vi "TDMS - AeroQuad File Viewer.vi"(4 "error in (no error)":errorcluster, 7 "file path":path) -> (0 "error out":errorcluster, 3 "file path out":path)   [LabVIEW 2010]
doc: "Opens the .tdms file specified in the <B>file path</B> input and presents the file data in the TDMS File Viewer dialog box."
uses:
  <vilib>/Utility/tdmsutil.llb/fileViewerConfigData.ctl
  <vilib>/Utility/error.llb/DialogType.ctl
  <vilib>/Utility/tdmsutil.llb/TDMSFileViewerLocalizedText.vi
  Instance           1 26Saved   TDMS - File Viewer .vi
panel:
  in  "Help":bool
  in  "Status":string
  in  "Quit":bool
  in  "Settings...":bool
  in  "Properties / Values / Graph":T1(tab)
  in  "Properties":i32(listbox)
  in  "Raw data values":i32(listbox)
  out "Waveform Graph":waveform(dbl)[](graph)
  in  "File contents":string(tree)
  # "Displaying values 1..1000"
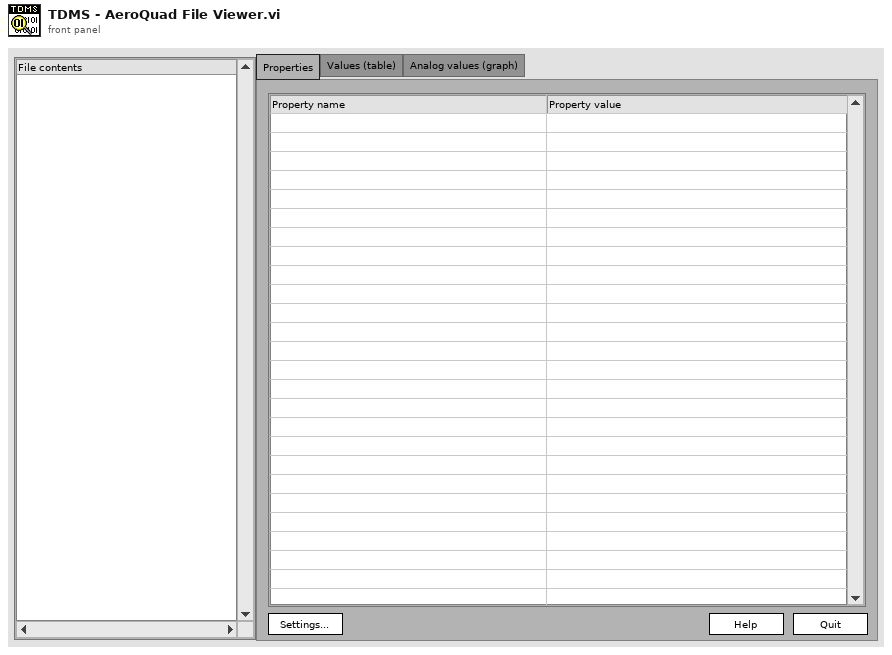
[diagram p1: front panel]
types:
  T1 = enum32{"Properties", "Values (table)", "Analog values (graph)"}
  T2 = enum16{"open", "open or create", "create or replace", "create", "open (read-only)"}
  T3 = typedef "fileViewerConfigData.ctl" = cluster{"Show all (table)":bool, "Show all (graph)":bool, "limit (table)":u64, "limit (graph)":u64, "no show":bool, "start (table)":u64, "start (graph)":u64}
  T4 = cluster{"Tree":refnum<vi>, "Tab Control":refnum<vi>, "property list":refnum<vi>, "raw data list":refnum<vi>, "Waveform Graph":refnum<vi>, "Ok":refnum<vi>, "Ok 2":refnum<vi>, "Ok 3":refnum<vi>, "Ok 4":refnum<vi>}
  T5 = typedef "LVRectTypeDef.ctl" = cluster{"left":i16, "top":i16, "right":i16, "bottom":i16}
  T6 = typedef "DialogType.ctl" = u16
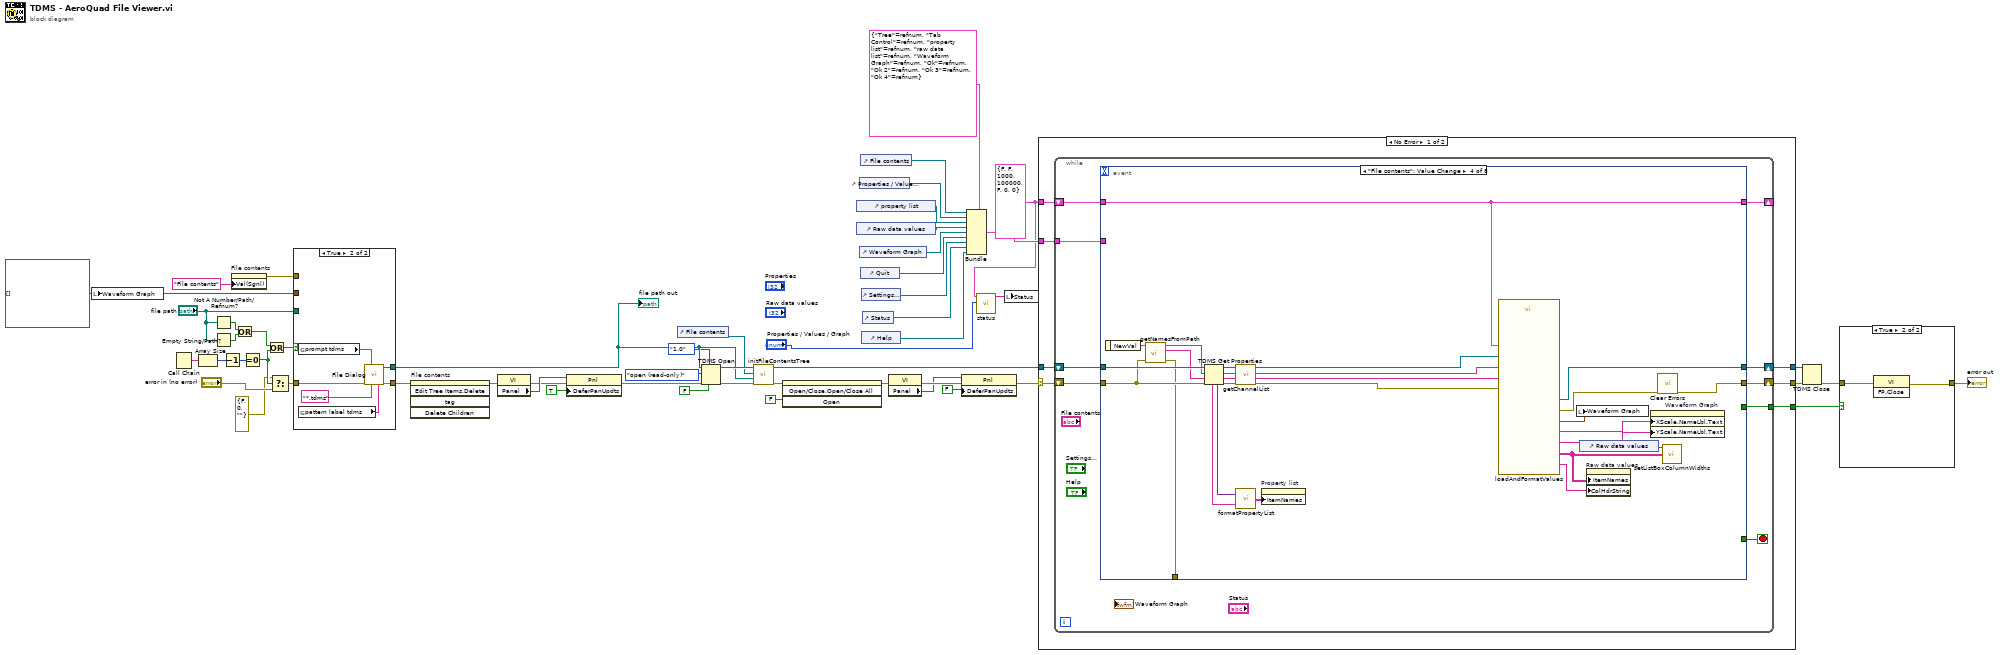
[diagram p0: block diagram]
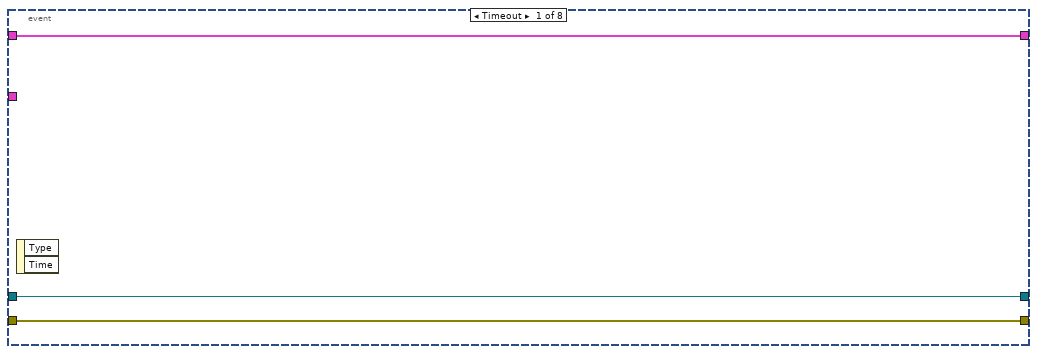
[diagram p3: hidden frame]
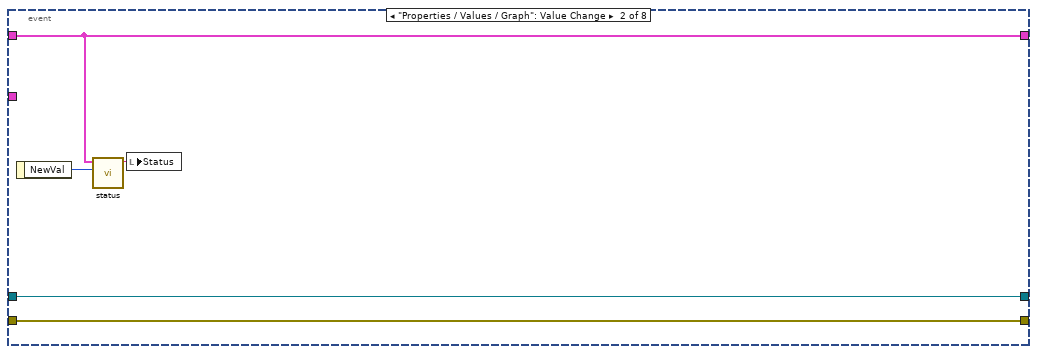
[diagram p4: hidden frame]
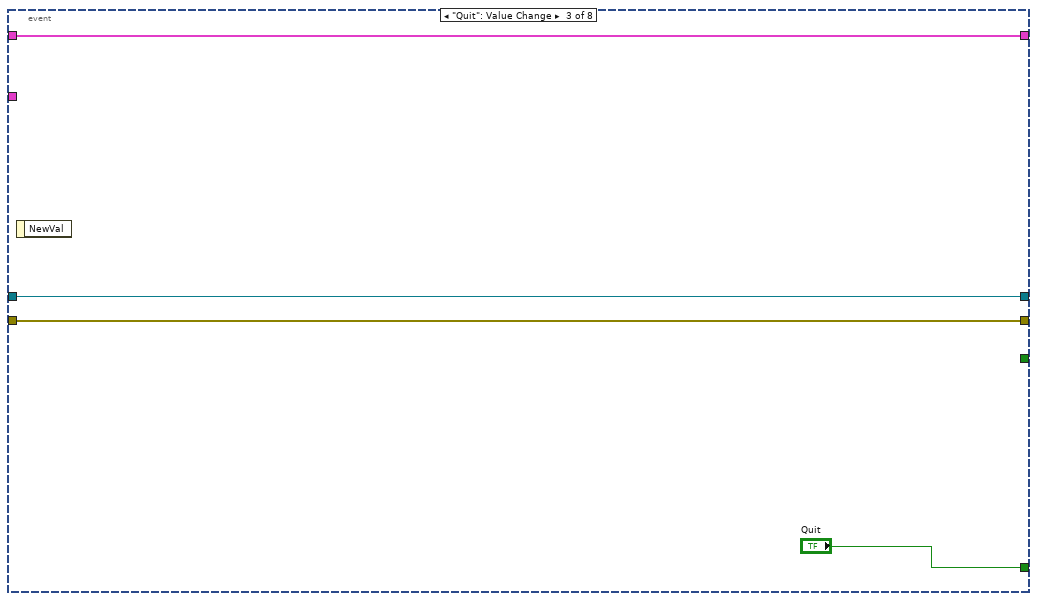
[diagram p5: hidden frame]
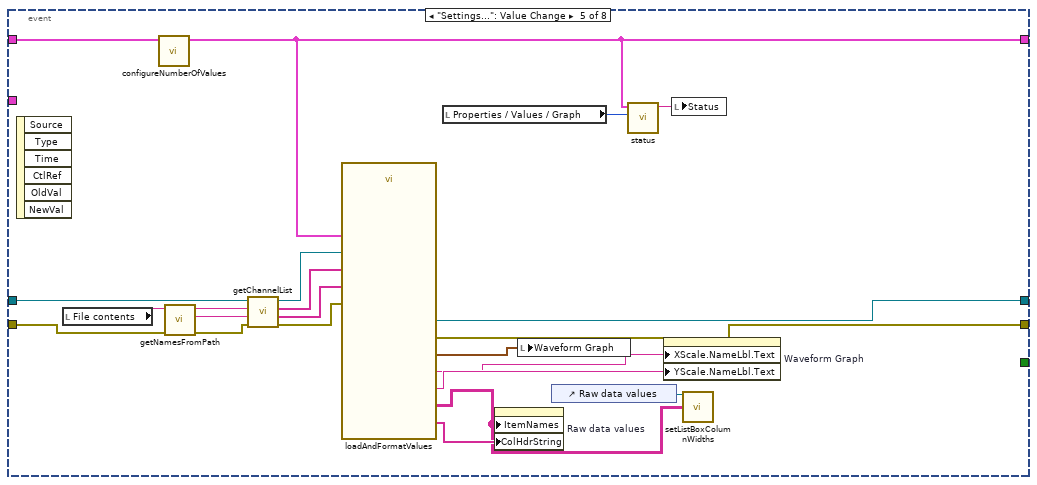
[diagram p6: hidden frame]
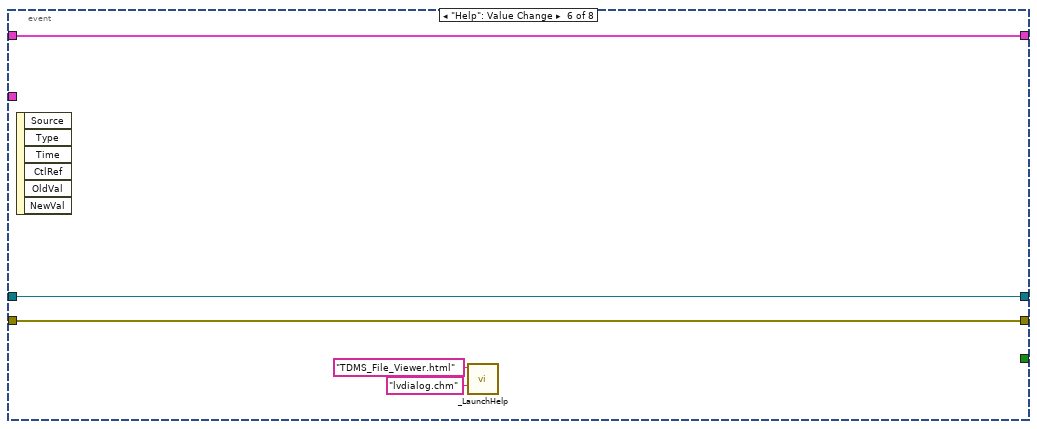
[diagram p7: hidden frame]
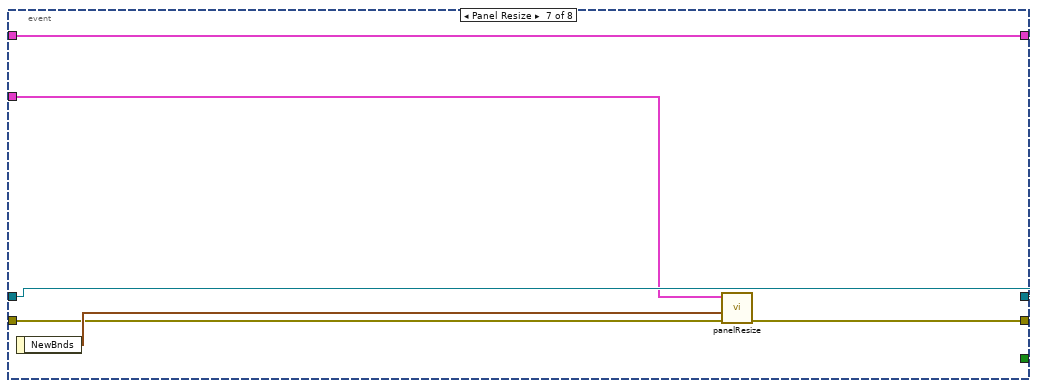
[diagram p8: hidden frame]
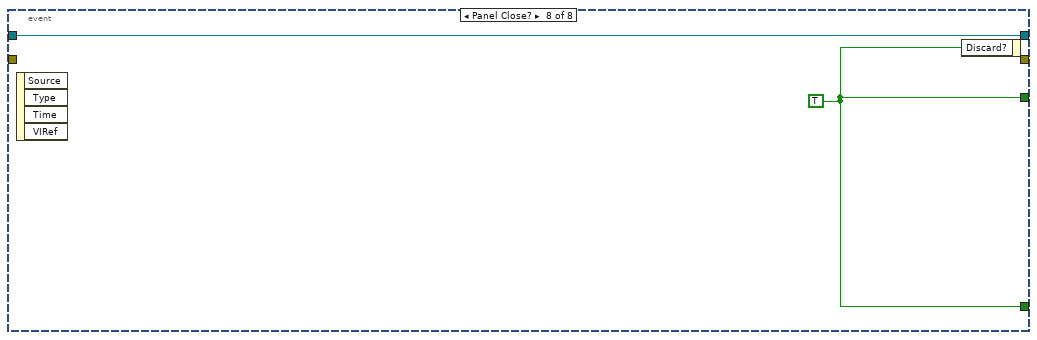
[diagram p9: hidden frame]
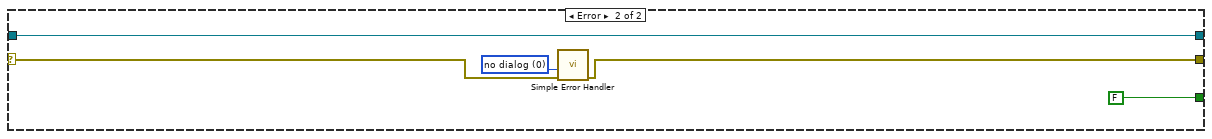
[diagram p10: hidden frame]
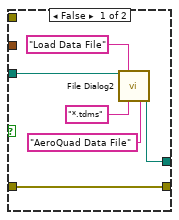
[diagram p11: hidden frame]
diagram:
  w1 = waveform(dbl)[] [] ("Waveform Graph")
  w15 = T3 {"Show all (table)"=FALSE, "Show all (graph)"=FALSE, "limit (table)"=1000, "limit (graph)"=100000, "no show"=FALSE, "start (table)"=0, "start (graph)"=0} ("TDMS File Viewer Configuration")
  n1 = local write "Waveform Graph"(w1) -> ()
  n2 = Call Chain() -> (call chain=w36:string[])
  n3 = Array Size(array=w36) -> (size(s)=w34:i32)
  n4 = Not A Number/Path/Refnum?(number/path/refnum="file path") -> (NaN/Path/Refnum?=w38:bool)
  n5 = Empty String/Path?(string/path="file path") -> (empty?=w37:bool)
  n6 = Decrement(x=w34) -> (x-1=w33:i32)
  n7 = property on="File contents" class="Tree (strict)"("Val(Sgnl)"="File contents" ("Value (Signaling)")) -> (error out=w2:errorcluster)  [unwired: 2 in, 1 out]
  n8 = Or(x=w38, y=w37) -> (x .or. y?=w35:bool)
  n9 = Equal To 0?(x=w33) -> (x = 0?=w13:bool)
  n10 = Or(x=w35, y=w13) -> (x .or. y?=w32:bool)
  n11 = Select(t=errorcluster {"status"=FALSE, "code"=0, "source"=""}, s=w13, f="error in (no error)") -> (s? t:f=w12:errorcluster)
  n12 = case shown="True" w32 {
    tunnel: [w59 w67] -> w20
    tunnel: "file path" -> [w60 _]
    tunnel: [w61 w65] -> w19
    tunnel: w12 -> [w61 w64]
    tunnel: w2 -> [_ _]
    tunnel: w1 -> [_ _]
    frame False {
      n13 = call "File Dialog2"("start path"=w60, "prompt"="Load Data File", "pattern (all files)"="*.tdms", "pattern label"="AeroQuad Data File") -> ("selected path"=w59:path)  [unwired: 8 in, 3 out]
    }
    frame True {
      n14 = global read "TDMSFileViewerLocalizedText.vi" "prompt tdms"() -> (w63:string)
      n15 = global read "TDMSFileViewerLocalizedText.vi" "pattern label tdms"() -> (w62:string)
      n16 = call "File Dialog"("prompt"=w63, "error in"=w64, "pattern (all files)"="*.tdms", "pattern label"=w62) -> ("selected path"=w67:path, "error out"=w65:errorcluster)  [unwired: 3 in, 7 out]
    }
  }
  "file path out" <- w20
  n17 = invoke on="File contents" class="Tree (strict)" method="Edit Tree Items.Delete"(error in=w19) -> (error out=w46:errorcluster)  [unwired: 4 in, 4 out]
  n18 = property class="VI"(error in=w46) -> (error out=w47:errorcluster, "Panel"=w48:refnum<vi>)  [unwired: 1 in, 1 out]
  n19 = property class="Pnl"(reference=w48, error in=w47, "DeferPanUpdts"=TRUE ("Defer Panel Updates")) -> (error out=w50:errorcluster)  [unwired: 1 out]
  n20 = control-ref of="File contents"() -> (w21:refnum<vi>)
  n21 = TDMS Open(6:FALSE ("disable buffering (T)"), 7:enum16{"1.0", "2.0"}."1.0" ("file format version (2.0)"), 8:w50, 10:T2."open (read-only)" ("operation"), 11:w20) -> (0:w55:errorcluster, 3:w54:refnum<k34>)  [unwired: 1 in]
  n22 = call <vilib>:"initFileContentsTree.vi"("error in (no error)"=w55, "file path"=w20, "Tree Refnum"=w21, "tdms file"=w54) -> ("error out"=w42:errorcluster, "tdms file out"=w53:refnum<k34>)  [unwired: 2 out]
  n23 = invoke on="File contents" class="Tree (strict)" method="Open/Close.Open/Close All"(error in=w42, "Open"=FALSE ("Open?")) -> (error out=w41:errorcluster)  [unwired: 2 in, 3 out]
  n24 = control-ref of="property list"() -> (w28:refnum<vi>)
  n25 = control-ref of="Raw data values"() -> (w27:refnum<vi>)
  n26 = control-ref of="Properties / Values / Graph"() -> (w29:refnum<vi>)
  n27 = control-ref of="Waveform Graph"() -> (w26:refnum<vi>)
  n28 = control-ref of="File contents"() -> (w31:refnum<vi>)
  n29 = control-ref of="Quit"() -> (w25:refnum<vi>)
  n30 = control-ref of="Settings..."() -> (w23:refnum<vi>)
  n31 = control-ref of="Help"() -> (w4:refnum<vi>)
  n32 = control-ref of="Status"() -> (w17:refnum<vi>)
  n33 = property class="VI"(error in=w41) -> (error out=w44:errorcluster, "Panel"=w43:refnum<vi>)  [unwired: 1 in, 1 out]
  n34 = property class="Pnl"(reference=w43, error in=w44, "DeferPanUpdts"=FALSE ("Defer Panel Updates")) -> (error out=w18:errorcluster)  [unwired: 1 out]
  n35 = Bundle(cluster=T4 {"Tree"=refnum, "Tab Control"=refnum, "property list"=refnum, "raw data list"=refnum, "Waveform Graph"=refnum, "Ok"=refnum, "Ok 2"=refnum, "Ok 3"=refnum, "Ok 4"=refnum} ("control refs"), "Tree"=w31, "Tab Control"=w29, "property list"=w28, "raw data list"=w27, "Waveform Graph"=w26, "Ok"=w25, "Ok 2"=w23, "Ok 3"=w17, "Ok 4"=w4) -> (w30:T4)
  n36 = call <vilib>:"status.vi"("tab sheet"="Properties / Values / Graph", "TDMS File Viewer Configuration"=w15) -> ("status"=w16:string)  [unwired: 5 out]
  n37 = local write "Status"(w16) -> ()
  n38 = case shown="No Error" w18 {
    selector: w18 -> [w69 w161]
    tunnel: w53 -> [w74 w162]
    tunnel: [w73 w162] -> w52
    tunnel: [w72 w160] -> w51
    tunnel: w30 -> [w71 _]
    tunnel: w15 -> [w70 _]
    tunnel: [w68 FALSE] -> w9
    frame No Error {
      n39 = while {
        shift-right: [w81] -> w72
        shift-left: w69 -> [w82]
        shift-right: [w80] -> w73
        shift-left: w74 -> [w83]
        tunnel: w71 -> [w78]
        shift-right: [w76] -> _
        shift-left: w70 -> [w77]
        tunnel: [w75] -> w68
        stop <- w79 stop-if-true
        n40 = event shown="[3] \"File contents\": Value Change" {
          selector: _ -> [_ _ _ _ _ _ _ _]
          dyn-events: _ -> [_ _ _ _ _ _ _ _]
          timeout: _ -> [_ _ _ _ _ _ _ _]
          tunnel: w83 -> [w85 w90 w94 w122 w133 w148 w155 w157]
          tunnel: w82 -> [w86 w91 w93 w114 w141 w147 w152 _]
          tunnel: [w86 w91 w93 w109 w142 w147 w151 _] -> w81
          tunnel: [w85 w90 w94 w121 w143 w148 w155 w157] -> w80
          tunnel: [_ _ "Quit" _ _ _ _ w156] -> w79
          tunnel: [_ _ _ w113 _ _ _ _] -> _
          tunnel: w78 -> [_ _ _ _ _ _ w153 _]
          tunnel: w77 -> [w84 w87 w92 w102 w144 w149 w150 _]
          tunnel: [w84 w87 w92 w102 w123 w149 w150 _] -> w76
          tunnel: [_ _ _ _ _ _ _ w156] -> w75
          event Timeout {
            n41 = event-data() -> ()  [unwired: 3 out]
          }
          event "Properties / Values / Graph": Value Change {
            n42 = event-data() -> ("NewVal"=w89:T1)  [unwired: 1 out]
            n43 = call <vilib>:"status.vi"("tab sheet"=w89, "TDMS File Viewer Configuration"=w87) -> ("status"=w88:string)  [unwired: 5 out]
            n44 = local write "Status"(w88) -> ()
          }
          event "Quit": Value Change {
            n45 = event-data() -> ()  [unwired: 2 out]
          }
          event "File contents": Value Change {
            n46 = event-data() -> ("NewVal"=w116:string)  [unwired: 1 out]
            n47 = call <vilib>:"getNamesFromPath.vi"("error in (no error)"=w114, "tree path"=w116) -> ("error out"=w113:errorcluster, "channel"=w119:string, "group"=w120:string)  [unwired: 3 out]
            n48 = TDMS Get Properties(8:w114, 9:w119, 10:w120, 11:w122) -> (0:w107:errorcluster, 1:w106:string, 2:w100:string, 3:w108:refnum<k34>, 4:w117:variant[], 6:w118:string[])  [unwired: 2 out]
            n49 = call <vilib>:"getChannelList.vi"("error in (no error)"=w107, "channel names"=w106, "group name"=w100, "tdms file"=w108) -> ("error out"=w96:errorcluster, "channel names out"=w97:string[], "group names out"=w98:string[], "tdms file out"=w99:refnum<k34>)
            n50 = call <vilib>:"formatPropertyList.vi"("property names"=w118, "property values"=w117) -> ("strings"=w115:string[][])
            n51 = property on="Property list" class="MCListbox (strict)"("ItemNames"=w115) -> ()  [unwired: 2 in, 2 out]
            n52 = call <vilib>:"loadAndFormatValues.vi"("error in (no error)"=w96, "configuration"=w102, "channel names"=w97, "group names"=w98, "tdms file"=w99) -> ("error out"=w110:errorcluster, "graph y names"=w104:string, "graph x names"=w103:string, "tdms file out"=w121:refnum<k34>, "waveform values"=w101:waveform(dbl)[], "table values"=w112:string[][], "table headers"=w105:string[])
            n53 = local write "Waveform Graph"(w101) -> ()
            n54 = control-ref of="Raw data values"() -> (w111:refnum<vi>)
            n55 = property on="Raw data values" class="MCListbox (strict)"("ItemNames"=w112, "ColHdrString"=w105) -> ()  [unwired: 2 in, 2 out]
            n56 = property on="Waveform Graph" class="WFGraph (strict)"("XScale.NameLbl.Text"=w103, "YScale.NameLbl.Text"=w104) -> ()  [unwired: 2 in, 2 out]
            n57 = call <vilib>:"Clear Errors.vi"("error in (no error)"=w110) -> ("error out"=w109:errorcluster)  [unwired: 6 out]
            n58 = call <vilib>:"setListBoxColumnWidths.vi"("table data"=w112, "MCListbox Refnum"=w111) -> ()  [unwired: 1 out]
          }
          event "Settings...": Value Change {
            n59 = event-data() -> ()  [unwired: 7 out]
            n60 = local read "File contents"() -> (w134:string)
            n61 = call <vilib>:"configureNumberOfValues.vi"("TDMS File Viewer Configuration"=w144) -> ("TDMS File Viewer Configuration Out"=w123:T3)  [unwired: 10 out]
            n62 = call <vilib>:"getNamesFromPath.vi"("error in (no error)"=w141, "tree path"=w134) -> ("error out"=w132:errorcluster, "channel"=w130:string, "group"=w131:string)  [unwired: 3 out]
            n63 = call <vilib>:"getChannelList.vi"("error in (no error)"=w132, "channel names"=w130, "group name"=w131, "tdms file"=w133) -> ("error out"=w129:errorcluster, "channel names out"=w126:string[], "group names out"=w127:string[], "tdms file out"=w128:refnum<k34>)
            n64 = call <vilib>:"loadAndFormatValues.vi"("error in (no error)"=w129, "configuration"=w123, "channel names"=w126, "group names"=w127, "tdms file"=w128) -> ("error out"=w142:errorcluster, "graph y names"=w136:string, "graph x names"=w135:string, "tdms file out"=w143:refnum<k34>, "waveform values"=w140:waveform(dbl)[], "table values"=w137:string[][], "table headers"=w139:string[])
            n65 = local read "Properties / Values / Graph"() -> (w124:T1)
            n66 = property on="Raw data values" class="MCListbox (strict)"("ItemNames"=w137, "ColHdrString"=w139) -> ()  [unwired: 2 in, 2 out]
            n67 = local write "Waveform Graph"(w140) -> ()
            n68 = control-ref of="Raw data values"() -> (w138:refnum<vi>)
            n69 = call <vilib>:"status.vi"("tab sheet"=w124, "TDMS File Viewer Configuration"=w123) -> ("status"=w125:string)  [unwired: 5 out]
            n70 = property on="Waveform Graph" class="WFGraph (strict)"("XScale.NameLbl.Text"=w135, "YScale.NameLbl.Text"=w136) -> ()  [unwired: 2 in, 2 out]
            n71 = local write "Status"(w125) -> ()
            n72 = call <vilib>:"setListBoxColumnWidths.vi"("table data"=w137, "MCListbox Refnum"=w138) -> ()  [unwired: 1 out]
          }
          event "Help": Value Change {
            n73 = event-data() -> ()  [unwired: 7 out]
            n74 = call <helpdir>:"_LaunchHelp.vi"("CHM or HLP filename (lvdialog.chm)"="lvdialog.chm", "HTML filename"="TDMS_File_Viewer.html") -> ()  [unwired: 1 in, 5 out]
          }
          event Panel Resize {
            n75 = event-data() -> ("NewBnds"=w154:T5)  [unwired: 1 out]
            n76 = call <vilib>:"panelResize.vi"("error in (no error)"=w152, "NewBnds"=w154, "control refs"=w153) -> ("error out"=w151:errorcluster)  [unwired: 4 out]
          }
          event Panel Close? {
            w156 = TRUE
            n77 = event-data() -> ()  [unwired: 5 out]
            n78 = event-data("Discard?"=w156) -> ()  [unwired: 1 in, 1 out]
          }
        }
      }
    }
    frame Error {
      w158 = T6 0 items=["no dialog", "OK message", "continue or stop message", "OK message + warnings", "continue/stop + warnings"] ("type of dialog (OK msg:1)")
      n79 = call <vilib>:"Simple Error Handler.vi"("type of dialog (OK msg:1)"=w158, "error in (no error)"=w161) -> ("error out"=w160:errorcluster)  [unwired: 7 out]
    }
  }
  n80 = TDMS Close(8:w51, 11:w52) -> (0:w8:errorcluster)  [unwired: 1 out]
  n81 = case shown="True" w9 {
    tunnel: w8 -> [w163 w165]
    tunnel: [w163 w164] -> w7
    frame False {
    }
    frame True {
      n82 = invoke class="VI" method="FP.Close"(error in=w165) -> (error out=w164:errorcluster)  [unwired: 2 in, 2 out]
    }
  }
  "error out" <- w7
